vi "Slerp.vi"(8 "error in":errorcluster, 9 "Sections":i32, 10 "End":dbl[](array[numeric]), 11 "Start":dbl[](array[numeric])) -> (0 "error out":errorcluster, 1 "Array":dbl[](array[numeric]), 3 "appended array":dbl[][](array[numeric]))   [LabVIEW 2011]
uses:
  <vilib>/Analysis/_algsub.llb/Real Vector Norm.vi
  <vilib>/Analysis/baseanly.llb/Real Dot Product.vi
  <vilib>/Analysis/NI_AALBase.lvlib
  <vilib>/Analysis/NI_AALPro.lvlib
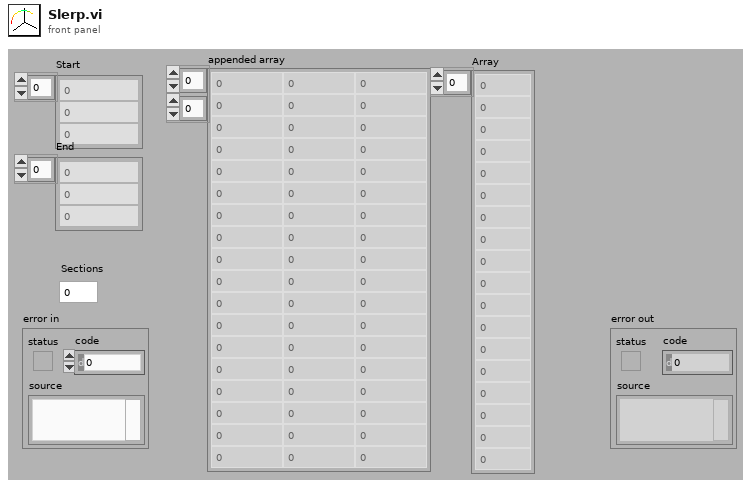
[diagram p1: front panel]
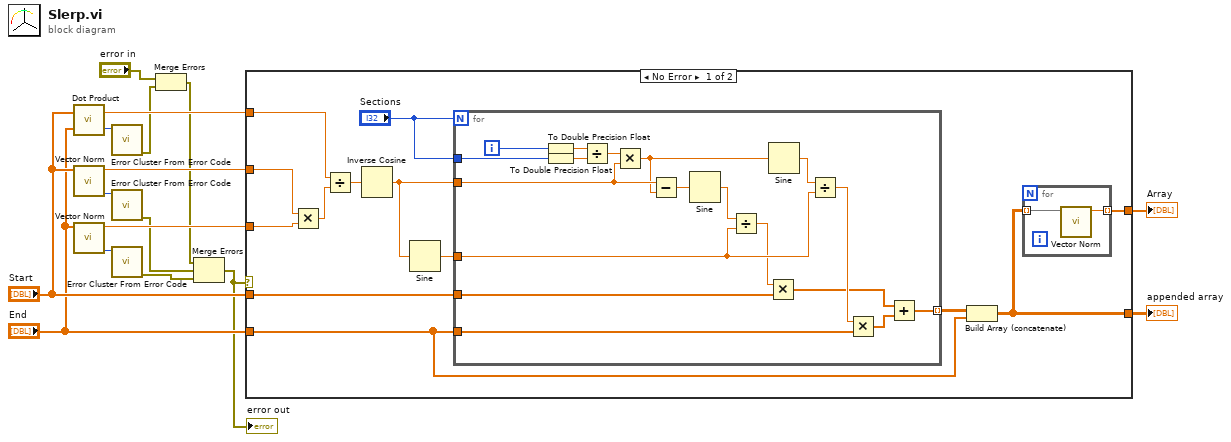
[diagram p0: block diagram]
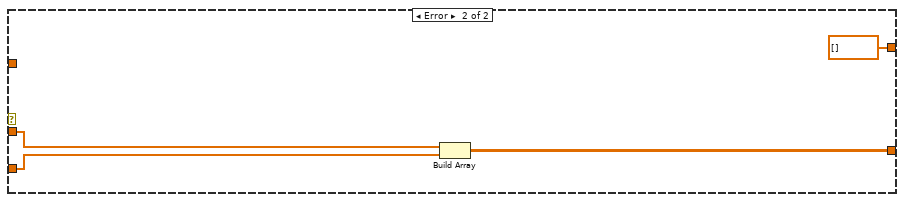
[diagram p2: hidden frame]
diagram:
  n1 = call-poly <vilib>:"Dot Product.vi"("Y Vector"="End", "X Vector"="Start") -> ("error"=w9:i32, "X * Y"=w14:dbl)
  n2 = call-poly <vilib>:"Vector Norm.vi"("Input Vector"="Start") -> ("error"=w8:i32, "norm"=w16:dbl)  [unwired: 9 in]
  n3 = call-poly <vilib>:"Vector Norm.vi"("Input Vector"="End") -> ("error"=w7:i32, "norm"=w15:dbl)  [unwired: 9 in]
  n4 = call <vilib>:"Error Cluster From Error Code.vi"("error code (0)"=w9) -> ("error out"=w2:errorcluster)  [unwired: 8 in]
  n5 = call <vilib>:"Error Cluster From Error Code.vi"("error code (0)"=w8) -> ("error out"=w5:errorcluster)  [unwired: 8 in]
  n6 = call <vilib>:"Error Cluster From Error Code.vi"("error code (0)"=w7) -> ("error out"=w6:errorcluster)  [unwired: 8 in]
  n7 = Merge Errors("error in", w2) -> (w1:errorcluster)
  n8 = Merge Errors(w1, w5, w6) -> (w4:errorcluster)
  "error out" <- w4
  n9 = case shown="No Error" w4 {
    tunnel: w16 -> [w29 _]
    tunnel: w15 -> [w28 _]
    tunnel: w14 -> [w27 _]
    tunnel: "Start" -> [w23 w52]
    tunnel: "End" -> [w19 w51]
    tunnel: [w18 w50] -> w11
    tunnel: [w17 dbl[] []] -> w10
    frame No Error {
      n10 = Multiply(x=w29, y=w28) -> (x*y=w26:dbl)
      n11 = Divide(x=w27, y=w26) -> (x/y=w25:dbl)
      n12 = Inverse Cosine(1:w25) -> (0:w24:dbl)
      n13 = Sine(x=w24) -> (sin(x)=w22:dbl)
      n14 = for {
        N: "Sections" -> [_]
        tunnel: w24 -> [w44]
        tunnel: w23 -> [w38]
        tunnel: w19 -> [w36]
        tunnel: w22 -> [w40]
        tunnel: "Sections" -> [w46]
        tunnel: [w33] -> w20 mode=indexing
        i -> [w32]
        n15 = To Double Precision Float(number=w32) -> (double precision float=w49:dbl)
        n16 = To Double Precision Float(number=w46) -> (double precision float=w48:dbl)
        n17 = Divide(x=w49, y=w48) -> (x/y=w47:dbl)
        n18 = Multiply(x=w47, y=w44) -> (x*y=w43:dbl)
        n19 = Subtract(x=w44, y=w43) -> (x-y=w42:dbl)
        n20 = Sine(x=w42) -> (sin(x)=w41:dbl)
        n21 = Divide(x=w41, y=w40) -> (x/y=w39:dbl)
        n22 = Multiply(x=w39, y=w38) -> (x*y=w34:dbl[])
        n23 = Sine(x=w43) -> (sin(x)=w45:dbl)
        n24 = Divide(x=w45, y=w40) -> (x/y=w37:dbl)
        n25 = Multiply(x=w37, y=w36) -> (x*y=w35:dbl[])
        n26 = Add(x=w34, y=w35) -> (x+y=w33:dbl[])
      }
      n27 = Build Array (concatenate)(w20, w19) -> (w18:dbl[][])
      n28 = for {
        tunnel: w18 -> [w31] mode=indexing
        tunnel: [w30] -> w17 mode=indexing
        n29 = call-poly <vilib>:"Vector Norm.vi"("Input Vector"=w31) -> ("norm"=w30:dbl)  [unwired: 9 in, 1 out]
      }
    }
    frame Error {
      n30 = Build Array(w52, w51) -> (w50:dbl[][])
    }
  }
  "appended array" <- w11
  "Array" <- w10
